vi "Update Gain Ranging Configuration.vi"(0 "session in":T2[](array[typedef]) {"rx baseband session"."3630 session"."Address Space" items=["VXI/VME A16"=1, "VXI/VME A24"=2, "VXI/VME A32"=3, "VXI/VME A64"=4, "PXI Memory Allocations"=9, "PXI Configuration"=10, "PXI BAR0"=11, "PXI BAR1"=12, "PXI BAR2"=13, "PXI BAR3"=14, "PXI BAR4"=15, "PXI BAR5"=16]; "tx baseband session"."3610 session"."Address Space" items=["VXI/VME A16"=1, "VXI/VME A24"=2, "VXI/VME A32"=3, "VXI/VME A64"=4, "PXI Memory Allocations"=9, "PXI Configuration"=10, "PXI BAR0"=11, "PXI BAR1"=12, "PXI BAR2"=13, "PXI BAR3"=14, "PXI BAR4"=15, "PXI BAR5"=16]}, 1 "scope":string(combo), 5 "coarse gain ranging entries":fxp<+/-,16,12>[](array[numeric])=[0.0, 0.0, 0.0, 0.0], 7 "gain config PXI triggers":string[](array[combo])=["None", "None"], 9 "mmWave port config PXI trigger":string(combo)="None", 11 "error in":errorcluster, 12 "enables":T1={"enable fine gain ranging"=TRUE, "enable coarse gain ranging"=TRUE, "enable port config"=TRUE}) -> (4 "session out":T2[](array[typedef]) {"rx baseband session"."3630 session"."Address Space" items=["VXI/VME A16"=1, "VXI/VME A24"=2, "VXI/VME A32"=3, "VXI/VME A64"=4, "PXI Memory Allocations"=9, "PXI Configuration"=10, "PXI BAR0"=11, "PXI BAR1"=12, "PXI BAR2"=13, "PXI BAR3"=14, "PXI BAR4"=15, "PXI BAR5"=16]; "tx baseband session"."3610 session"."Address Space" items=["VXI/VME A16"=1, "VXI/VME A24"=2, "VXI/VME A32"=3, "VXI/VME A64"=4, "PXI Memory Allocations"=9, "PXI Configuration"=10, "PXI BAR0"=11, "PXI BAR1"=12, "PXI BAR2"=13, "PXI BAR3"=14, "PXI BAR4"=15, "PXI BAR5"=16]}, 6 "coerced coarse gain ranging entries":dbl[](array[numeric]), 15 "error out":errorcluster)   [LabVIEW 2019]
uses:
  TypeDefs/Session.ctl
  <instrlib>/niMmWave/ni3620/Config/v1/Host/Public/High-Level/niMmWave Session.ctl
  <instrlib>/_niInstr/Register Bus/v0/Host/Public/Register Bus Session.ctl
  <instrlib>/_niInstr/Register Bus/v0/Host/Private/Session Data.ctl
  <instrlib>/niMmWave/ni3620/Config/v1/Host/Public/Typedefs/Board Information.ctl
  <instrlib>/niMmWave/ni3620/Config/v1/Host/Public/Typedefs/Hardware Revision.ctl
  <instrlib>/niMmWave/ni3620/Config/v1/Host/Public/Typedefs/Gain Mapping.ctl
  <instrlib>/niMmWave/ni3620/Config/v1/Host/Public/Typedefs/Correction Data.ctl
  <instrlib>/niMmWave/ni3620/Config/v1/Host/Public/Typedefs/Opera Characterization.ctl
  <instrlib>/niMmWave/ni3620/Config/v1/Host/Public/Corrections/Typedefs/Opera Characterization Main Header.ctl
  <instrlib>/niMmWave/ni3620/Config/v1/Host/Public/Corrections/Typedefs/Opera IF Board Information.ctl
  <instrlib>/niMmWave/ni3620/Config/v1/Host/Public/Corrections/Typedefs/Opera Characterization Instance Header.ctl
  <instrlib>/niMmWave/ni3620/Config/v1/Host/Public/Corrections/Typedefs/Opera Characterization Device Data Header.ctl
  <instrlib>/niMmWave/ni3620/Config/v1/Host/Public/Corrections/Typedefs/Opera LO Characterization Data Header.ctl
  <instrlib>/niMmWave/ni3620/Config/v1/Host/Public/Corrections/Typedefs/Opera IF Board Characterization Data Header.ctl
  <instrlib>/niMmWave/ni3620/Config/v1/Host/Public/Corrections/Typedefs/Opera Characterization Device Data.ctl
  <instrlib>/niMmWave/ni3620/Config/v1/Host/Public/Corrections/Typedefs/Opera LO2 Board Characterization Data.ctl
  <instrlib>/niMmWave/ni3620/Config/v1/Host/Public/Corrections/Typedefs/Opera LO Characterization Data.ctl
  <instrlib>/niMmWave/ni3620/Config/v1/Host/Public/Corrections/Typedefs/Opera IF Board Characterization Data.ctl
  <instrlib>/niMmWave/ni3620/Config/v1/Host/Public/Corrections/Typedefs/Opera IQ Impairment Data.ctl
  <instrlib>/niMmWave/ni3620/Config/v1/Host/Public/Typedefs/mmWave Adapter Session Data.ctl
  <instrlib>/niMmWave/ni3620/Config/v1/Host/Public/Typedefs/mmWave Adapter Data.ctl
  <instrlib>/niMmWave/ni3620/Config/v1/Host/Public/Typedefs/mmWave Adapter 2.ctl
  <instrlib>/niMmWave/ni3620/Config/v1/Shared/Typedefs/Subsystem ID.ctl
  <instrlib>/niMmWave/ni3620/Config/v1/Host/Public/Typedefs/mmWave Adapter Channel Information.ctl
  <instrlib>/niMmWave/ni3620/Config/v1/Host/Public/Typedefs/Temperature Coefficients.ctl
  <instrlib>/niMmWave/ni3620/Config/v1/Host/Public/Typedefs/mmWave Characterization.ctl
  <instrlib>/niMmWave/ni3620/Config/v1/Host/Public/Corrections/Typedefs/mmWave Characterization Main Header.ctl
  <instrlib>/niMmWave/ni3620/Config/v1/Host/Public/Corrections/Typedefs/mmWave Characterization Instance Header.ctl
  <instrlib>/niMmWave/ni3620/Config/v1/Host/Public/Typedefs/Session Cache.ctl
  <instrlib>/niMmWave/ni3620/Config/v1/Host/Public/Typedefs/LO2 settings cache.ctl
  <instrlib>/niMmWave/ni3620/Config/v1/Host/Public/Typedefs/LO2 source.ctl
  <instrlib>/niMmWave/ni3620/Config/v1/Host/Public/Typedefs/Desired and Coerced.ctl
  <instrlib>/niMmWave/ni3620/Config/v1/Host/Public/Typedefs/Export cache.ctl
  <instrlib>/niMmWave/ni3620/Config/v1/Host/Public/Typedefs/Path cache.ctl
  <instrlib>/niMmWave/ni3620/Config/v1/Host/Public/Typedefs/Daughterboard Type.ctl
  <instrlib>/niMmWave/ni3620/Config/v1/Host/Public/Typedefs/LO1 settings cache.ctl
  <instrlib>/niMmWave/ni3620/Config/v1/Host/Public/Typedefs/LO1 Source.ctl
  <instrlib>/niMmWave/ni3620/Config/v1/Host/Public/Typedefs/mmWave export cache.ctl
  <instrlib>/niMmWave/ni3620/Config/v1/Host/Private/Board/LO2/LO2 Board Configuration Cache.ctl
  <instrlib>/niMmWave/ni3620/Config/v1/Host/Public/Typedefs/reference clock routing settings.ctl
  <instrlib>/niMmWave/ni3620/Config/v1/Host/Public/Typedefs/LO2 routing settings.ctl
  <instrlib>/niMmWave/ni3620/Config/v1/Host/Private/Board/LO1/LO1 Board Configuration Cache.ctl
  <instrlib>/niMmWave/ni3620/Config/v1/Host/Public/Typedefs/LO1 source settings.ctl
  <instrlib>/niMmWave/ni3620/Config/v1/Host/Public/Typedefs/LO1 export settings.ctl
  <instrlib>/niMmWave/ni3620/Config/v1/Host/Public/Typedefs/LO1 mmWave settings.ctl
  TypeDefs/Tx Baseband Session.ctl
  <instrlib>/niMmWave/ni3610 and ni3630/controls/public/Main Settings.ctl
  <vilib>/Instr/_visa.llb/VISA Register Access Address Space.ctl
  <instrlib>/niMmWave/ni3610 and ni3630/controls/public/Register Adresses.ctl
  <instrlib>/niMmWave/ni3610 and ni3630/controls/public/Base Card Type.ctl
  <instrlib>/niMmWave/ni3610 and ni3630/controls/private/IQ Card Revision.ctl
  <instrlib>/niMmWave/ni3610 and ni3630/controls/public/Board Capability.ctl
  TypeDefs/Blank FPGA Reference.ctl
  TypeDefs/Rx Baseband Session.ctl
  TypeDefs/Hardware Configuration.ctl
  TypeDefs/Direction.ctl
  TypeDefs/Gain Ranging.ctl
  TypeDefs/PXI Trigger Bus Info.ctl
  TypeDefs/Gain Ranging Reference.ctl
  <vilib>/rvi/errors/niLvFpgaAdjustHostInterfaceError.vi
  <vilib>/rvi/interface/nirviReadWriteControl/nirviReadWriteControl.xnode
  <instrlib>/niMmWave/ni3620/Config/v1/Host/niMmWave Config v1 Host.lvlib
  NiFpgaLv.dll
  <vilib>/rvi/interface/Simulation/niFpgaSimulationCallBeginRW.vi
  <instrlib>/_niInstr/Register Bus/v0/Host/niInstr Register Bus v0 Host.lvlib
  <instrlib>/niMmWave/ni3610 and ni3630/ni3610_and_ni3630_Driver_Lib.lvlib
  <instrlib>/niMmWave/ni3620/Config/v1/Shared/niMmWave Config v1 Shared.lvlib
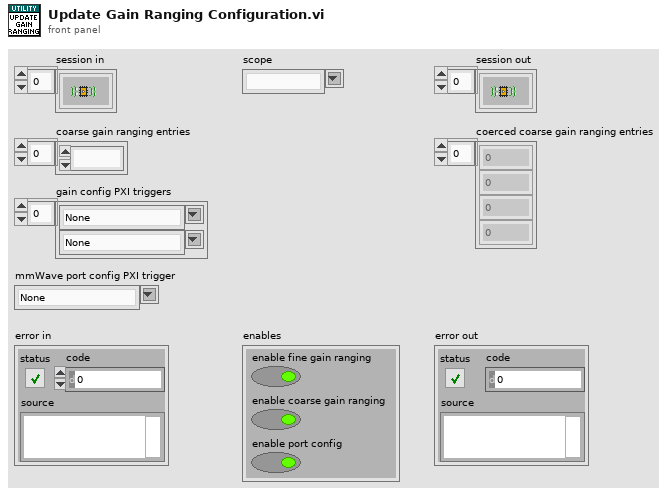
[diagram p1: front panel]
types:
  T1 = cluster{"enable fine gain ranging":bool, "enable coarse gain ranging":bool, "enable port config":bool}
  T2 = typedef "Session.ctl" = cluster{"3620 session":refnum<queue>, "tx baseband session":T3, "rx baseband session":T11, "tx gain (dB)":dbl, "rx gain (dB)":dbl, "hardware configuration":T12, "gain ranging":T14[], "pxi trigger bus information":T15}
  T3 = typedef "Tx Baseband Session.ctl" = cluster{"3610 session":T4, "7902 reference":T10}
  T4 = typedef "ni3610_and_ni3630_Driver_Lib.lvlib/Main Settings.ctl" = cluster{"VISA resource name":refnum<visa-resource-name>, "Address Space":T5, "window_offset":u32, "register_addresses":T6, "required_MM_fpga_version":cluster{"signature":u32, "hardware":u32, "current revision":u32, "oldest revision":u32}, "CPLD Oldest Compat Version ":cluster{"hardware":u32, "CPLD firmware":u32}, "MM_FPGA_image_location":string, "is_init":bool, "card_type":T7, "DacLmkConfigFileName":string, "AdcLmkConfigFileName":string, "AdcConfigFileName":string, "DacConfigFileName_RevA":string, "DacConfigFileName_RevB":string, "Mulde hardware revision":u8, "bypass DAC PLL\n":bool, "IQ Card Revision":T8, "board capability":T9}
  T5 = typedef "VISA Register Access Address Space.ctl" = u16
  T6 = typedef "ni3610_and_ni3630_Driver_Lib.lvlib/Register Adresses.ctl" = cluster{"MM based Registers":cluster{"Revision":u32, "OldestCompatRev":u32, "signature":u32, "scratch":u32, "LedControl":u32, "BoardHwRev":u32, "BoardControl":u32, "ThermalStatus":u32, "BasebandStatus":u32, "BasebandControl":u32, "BasebandAuxSetup":u32, "BasebandAuxStatus":u32, "LmkSyncOutSetup":u32, " AdcSyncOutSetup":u32, " InjSyncOutSetup":u32, " PxiTrig0OutSetup":u32, " PxiTrig1OutSetup":u32, " PxiTrig2OutSetup":u32, " PxiTrig3OutSetup":u32, " PxiTrig4OutSetup":u32, " PxiTrig5OutSetup":u32, " PxiTrig6OutSetup":u32, " PxiTrig7OutSetup":u32}, "CPLD based Registers":cluster{"SlaveSignature":u32, "SlaveRevision":u32, "SlaveOldestCompatRev":u32, "SlaveScratch":u32, "SlaveSetup":u32, "SlaveStatus":u32, "IDacReg_offset":u32, "LMKRegGrp0_offset":u32, "QDacReg_offset":u32, "BrdTempSensorVal":u32, "TempSensorPowerDown":u32, "GPIOReg_offset":u32, "IAdcReg_offset":u32, "QAdcReg_offset":u32, "LMKRegGrp1_offset":u32, "QadcTempSensorVal":u32, "IadcTempSensorVal":u32, "RevisionReg":u32, "VcxoReg":u32, "CpldStatusReg":u32, "PowerReg":u32, "VBiasEnReg":u32, "ExtRefOeReg":u32, "QdacCtrlReg":u32, "QdacStatusReg":u32, "IdacCtrlReg":u32, "IdacStatusReg":u32, "QdacJtagIn":u32, "QdacJtagOut":u32, "IdacJtagIn":u32, "IdacJtagOut":u32, "IqDcSetupReg":u32, "QadcStatusReg":u32, "IadcStatusReg":u32, "BrdSetupReg":u32, "IqDcRevisionReg":u32, "PllStatusReg":u32, "EndpointScratchReg":u32, "AdcSyncCfgReg":u32, "IqCardOpampReg":u32}, "CPLD Register Offset":u32, "MM  Register Offset":u32, " PxiTrig0OutSetup":u32}
  T7 = typedef "ni3610_and_ni3630_Driver_Lib.lvlib/Base Card Type.ctl" = enum16{"unspecified", "ADC", "DAC"}
  T8 = typedef "ni3610_and_ni3630_Driver_Lib.lvlib/IQ Card Revision.ctl" = enum16{"RevA", "RevB", "RevC", "RevD"}
  T9 = typedef "ni3610_and_ni3630_Driver_Lib.lvlib/Board Capability.ctl" = cluster{"baseband sync":enum16{"no baseband sync", "baseband sync"}}
  T10 = typedef "Blank FPGA Reference.ctl" = refnum<k20>
  T11 = typedef "Rx Baseband Session.ctl" = cluster{"3630 session":T4, "7902 reference":T10}
  T12 = typedef "Hardware Configuration.ctl" = cluster{"direction":T13, "baseband only":bool}
  T13 = typedef "Direction.ctl" = enum16{"Transceiver", "Receiver", "Transmitter"}
  T14 = typedef "Gain Ranging.ctl" = cluster{"gain ranging active scope":string, "gain ranging stream session":refnum<k20>}
  T15 = typedef "PXI Trigger Bus Info.ctl" = cluster{"chassis resource name":refnum<visa-resource-name>, "7902R (TX)":i16, "3610 (TX)":i16, "3620 (IF)":i16, "3630 (RX)":i16, "7902R (RX)":i16}
  T16 = typedef "Gain Ranging Reference.ctl" = refnum<k20>
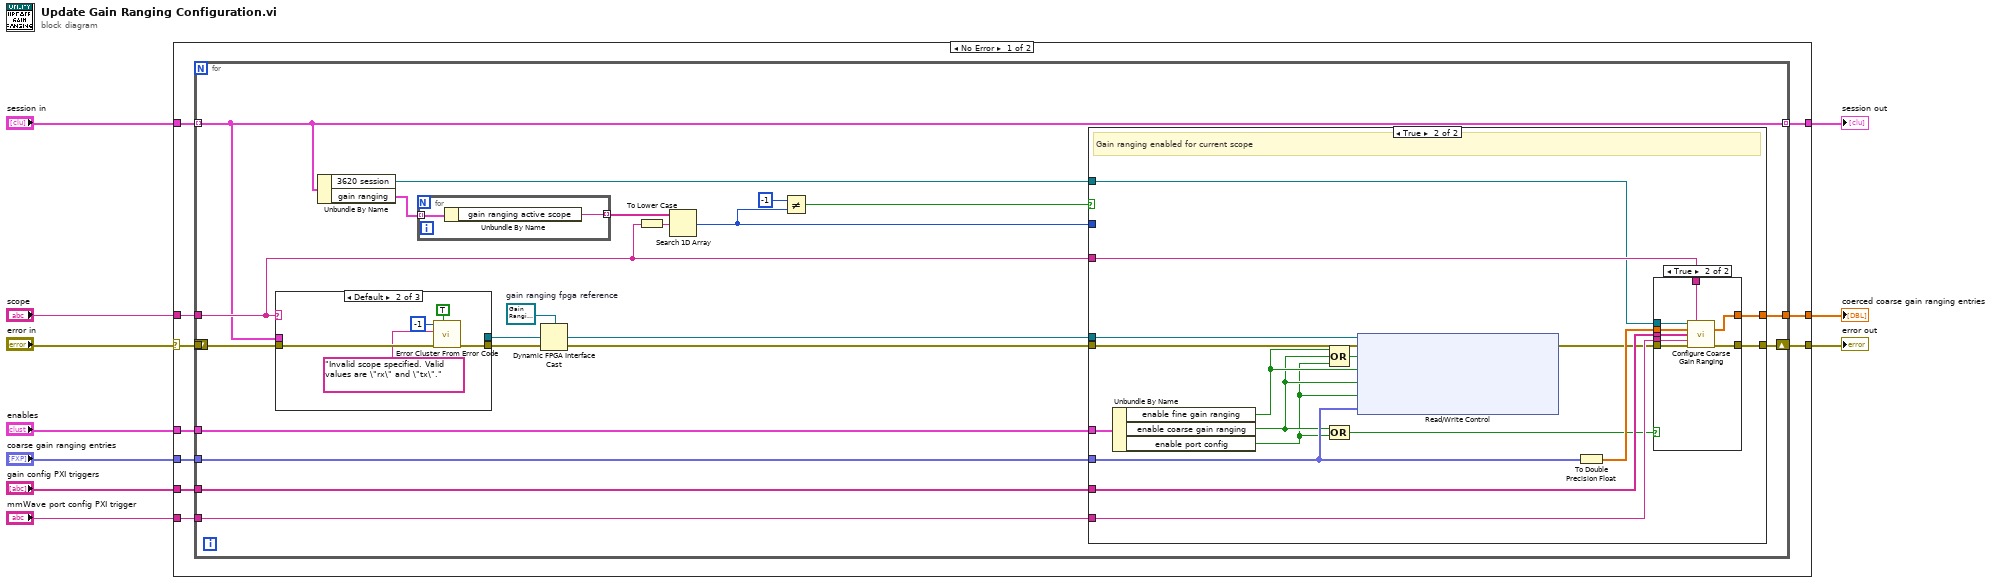
[diagram p0: block diagram]
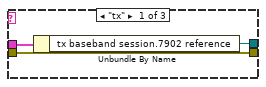
[diagram p2: hidden frame]
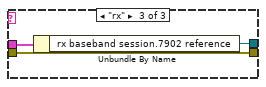
[diagram p3: hidden frame]
diagram:
  n1 = case shown="No Error" "error in" {
    selector: "error in" -> [w16 w82]
    tunnel: [w20 w82] -> w10
    tunnel: "session in" -> [w19 w81]
    tunnel: "scope" -> [w18 _]
    tunnel: [w17 w81] -> w7
    tunnel: "coarse gain ranging entries" -> [w15 _]
    tunnel: "gain config PXI triggers" -> [w14 _]
    tunnel: [w13 _] -> w4
    tunnel: "mmWave port config PXI trigger" -> [w12 _]
    tunnel: "enables" -> [w11 _]
    frame No Error {
      n2 = for {
        shift-right: [w39] -> w20
        shift-left: w16 -> [w35]
        tunnel: w19 -> [w21] mode=indexing
        tunnel: w18 -> [w29]
        tunnel: [w21] -> w17 mode=indexing
        tunnel: w16 -> [_]
        tunnel: w15 -> [w28]
        tunnel: w14 -> [w27]
        tunnel: [w26] -> w13
        tunnel: w12 -> [w25]
        tunnel: w11 -> [w22]
        w38 = T16 refnum  # gain ranging fpga reference
        n3 = case shown="Default" w29 {
          tunnel: [w43 w49 w53] -> w23
          tunnel: w35 -> [w43 w50 w53]
          tunnel: w21 -> [w45 _ w52]
          tunnel: [w44 _ w51] -> w37
          frame "tx" {
            n4 = Unbundle By Name(w45) -> ("tx baseband session.7902 reference"=w44:T10)
          }
          frame Default {
            n5 = call <vilib>:"Error Cluster From Error Code.vi"("show call chain? (False)"=TRUE, "error in (no error)"=w50, "error message (\"\")"="Invalid scope specified. Valid values are \"rx\" and \"tx\"." ("error message (\"\")"), "error code (0)"=-1) -> ("error out"=w49:errorcluster)  [unwired: 5 in]
          }
          frame "rx" {
            n6 = Unbundle By Name(w52) -> ("rx baseband session.7902 reference"=w51:T10)
          }
        }
        n7 = Unbundle By Name(w21) -> ("3620 session"=w36:refnum<queue>, "gain ranging"=w32:T14[])
        n8 = for {
          tunnel: w32 -> [w42] mode=indexing
          tunnel: [w41] -> w34 mode=indexing
          n9 = Unbundle By Name(w42) -> ("gain ranging active scope"=w41:string)
        }
        n10 = Dynamic FPGA Interface Cast(Session In=w38, Type=w37) -> (Session Out=w40:T16)
        n11 = To Lower Case(string=w29) -> (all lower case string=w33:string)
        n12 = Search 1D Array(1D array=w34, element=w33) -> (index of element=w30:i32)  [unwired: 1 in]
        n13 = Not Equal?(x=-1, y=w30) -> (x != y?=w24:bool)
        n14 = case shown="True" w24 {
          tunnel: w40 -> [_ w71]
          tunnel: [w54 w62] -> w39
          tunnel: w23 -> [w54 w70]
          tunnel: w36 -> [_ w63]
          tunnel: w29 -> [_ w69]
          tunnel: w30 -> [_ _]
          tunnel: w28 -> [_ w68]
          tunnel: w27 -> [_ w67]
          tunnel: [_ w66] -> w26
          tunnel: w25 -> [_ w65]
          tunnel: w22 -> [_ w61]
          frame False {
            # "Gain ranging disabled for current scope. Do nothing"
          }
          frame True {
            # "Gain ranging enabled for current scope"
            n15 = Unbundle By Name(w61) -> ("enable fine gain ranging"=w59:bool, "enable coarse gain ranging"=w57:bool, "enable port config"=w56:bool)
            n16 = Compound Arithmetic op=OR(w59, w57, w56) -> (w58:bool)
            n17 = Compound Arithmetic op=OR(w57, w56) -> (w55:bool)
            n18 = xnode "Read/Write Control"("FPGA VI Reference In"=w71, "error in"=w70, "gain ranging.enable"=w58, "gain ranging.enable fine gain ranging"=w59, "gain ranging.enable coarse gain ranging"=w57, "gain ranging.enable port config"=w56, "gain ranging.coarse gain values"=w68) -> ("error out"=w60:errorcluster)  [unwired: 1 out]
            n19 = To Double Precision Float(number=w68) -> (double precision float=w64:dbl[])
            n20 = case shown="True" w55 {
              tunnel: w69 -> [_ w80]
              tunnel: w67 -> [_ w79]
              tunnel: [_ w78] -> w66
              tunnel: w65 -> [_ w77]
              tunnel: w64 -> [_ w76]
              tunnel: w63 -> [_ w75]
              tunnel: w60 -> [w72 w74]
              tunnel: [w72 w73] -> w62
              frame False {
              }
              frame True {
                n21 = call <instrlib>:"Configure Coarse Gain Ranging.vi"("session in"=w75, "scope"=w80, "coarse gain ranging entries [4]"=w76, "gain config PXI triggers [2]"=w79, "mmWave port config PXI trigger"=w77, "error in"=w74) -> ("coerced coarse gain ranging entries"=w78:dbl[], "error out"=w73:errorcluster)  [unwired: 7 in, 1 out]
              }
            }
          }
        }
      }
    }
    frame Error {
    }
  }
  "error out" <- w10
  "session out" <- w7
  "coerced coarse gain ranging entries" <- w4
